vi "SPI read.vi"(6 "Number of bytes":i32=1, 8 "error in (no error)":errorcluster, 9 "Address":u8, 10 "spi configuration in":T2, 11 "Device ref in":T1) -> (0 "error out":errorcluster, 1 "read data":u8[](array[numeric]), 2 "spi configuration out":T2, 3 "Device ref out":T1)   [LabVIEW 2013]
uses:
  <vilib>/ni845x/ni845x.llb/ni845xSpiConfiguration.ctl
  <vilib>/ni845x/ni845x.llb/ni845xControl.ctl
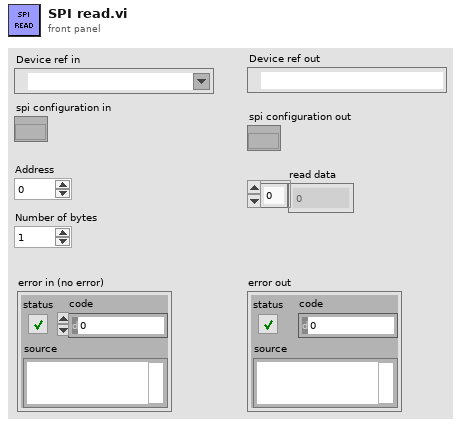
[diagram p1: front panel]
types:
  T1 = typedef "ni845xControl.ctl" = refnum<k21>
  T2 = typedef "ni845xSpiConfiguration.ctl" = refnum<k20>
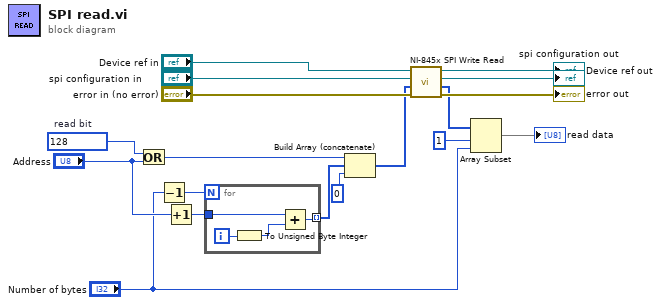
[diagram p0: block diagram]
diagram:
  w11 = u8 128  # read bit
  n1 = Or(x=w11, y="Address") -> (x .or. y?=w8:u8)
  n2 = Decrement(x="Number of bytes") -> (x-1=w9:i32)
  n3 = Increment(x="Address") -> (x+1=w10:u8)
  n4 = for {
    N: w9 -> [_]
    tunnel: w10 -> [w22]
    tunnel: [w21] -> w7 mode=indexing
    i -> [w20]
    n5 = To Unsigned Byte Integer(number=w20) -> (unsigned 8bit integer=w19:u8)
    n6 = Add(x=w22, y=w19) -> (x+y=w21:u8)
  }
  n7 = Build Array (concatenate)(w8, w7, u8 0 ("element")) -> (w5:u8[])
  n8 = call <vilib>:"NI-845x SPI Write Read.vi"("error in (no error)"="error in (no error)", "write data"=w5, "spi configuration in"="spi configuration in", "device reference in"="Device ref in") -> ("error out"=→"error out":errorcluster, "read data"=w4:u8[], "spi configuration out"=→"spi configuration out":T2, "device reference out"=→"Device ref out":T1)  [unwired: 4 in]
  n9 = Array Subset(array=w4, index=1, length="Number of bytes") -> (→"read data":u8[])
